vi "Read Array of TA Binding.vi"(11 "Motions in":refnum<class "Motions.lvclass">) -> (2 "Array of TA Binding":T1[](array[typedef]), 3 "Motions out":refnum<class "Motions.lvclass">)   [LabVIEW 2016, in "Hardware.lvlib" / "Motions.lvlib" / "Motions.lvclass"]
uses:
  <userlib>/Common Components/Hardware/Abstract System/Motions/Motions/Motions.lvclass
  <userlib>/Common Components/Hardware/Abstract System/Motions/Motions/TA Binding Data.ctl
  <userlib>/Common Components/Hardware/Abstract System/Motions/Motions/Motions.lvclass/Motions.ctl
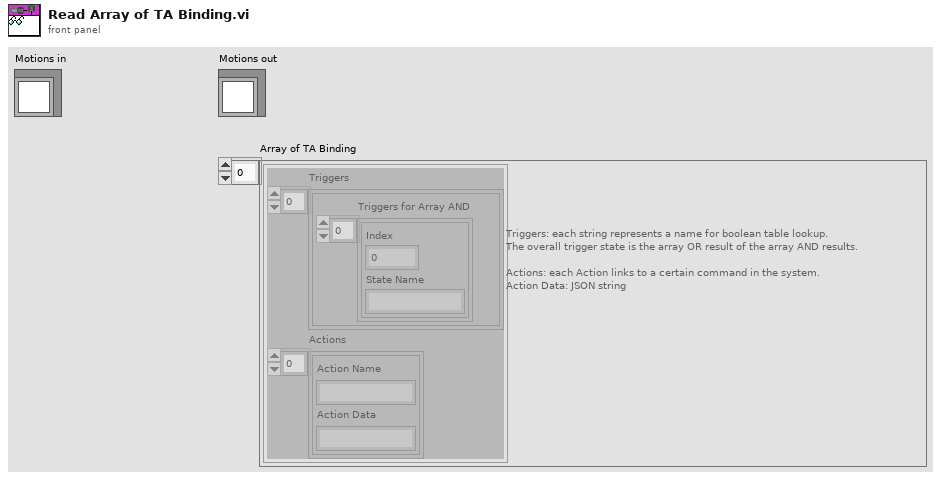
[diagram p1: front panel]
types:
  T1 = typedef "Hardware.lvlib/Motions.lvlib/Motions.lvclass/TA Binding Data.ctl" = cluster{"Triggers":cluster{"Triggers for Array AND":cluster{"Index":u8, "State Name":string}[]}[], "Actions":cluster{"Action Name":string, "Action Data":string}[]}
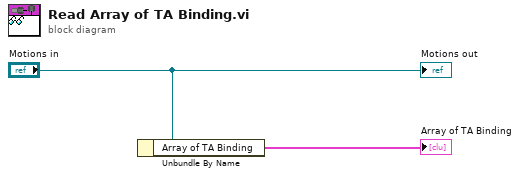
[diagram p0: block diagram]
diagram:
  n1 = Unbundle By Name("Motions in") -> ("Array of TA Binding"=→"Array of TA Binding":T1[])
  "Motions out" <- "Motions in"
